vi "Step Output.vi"(8 "error in (no error)":errorcluster, 11 "IV in":refnum<class "IV.lvclass">) -> (0 "error out":errorcluster, 3 "IV out":refnum<class "IV.lvclass">)   [LabVIEW 2021, in "IV.lvclass"]
uses:
  IV.lvclass
  Libraries/Utilities/Output Value/Output Value.lvclass
  C:/Git/NHMFL_Core/Libraries/Instruments/Results/Acquired Result/Acquired Result.lvclass
  Libraries/Instruments/Instrument Driver/Instrument Driver.lvclass
  IV.lvclass/IV.ctl
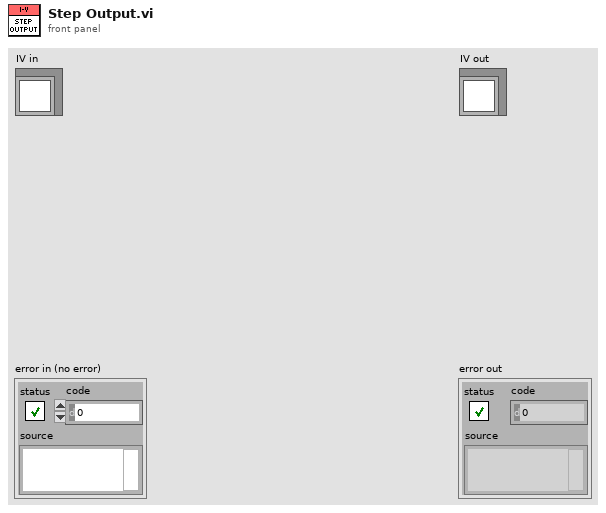
[diagram p1: front panel]
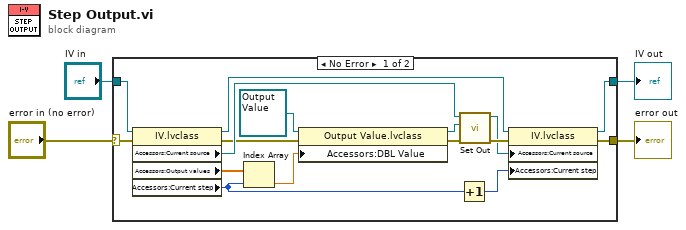
[diagram p0: block diagram]
diagram:
  n1 = case shown="No Error" "error in (no error)" {
    selector: "error in (no error)" -> [w20 w22]
    tunnel: [w14 w22] -> w3
    tunnel: [w12 w21] -> w1
    tunnel: "IV in" -> [w19 w21]
    frame No Error {
      n2 = property class="IV.lvclass"(reference=w19, error in=w20) -> (reference out=w13:refnum<class "IV.lvclass">, error out=w8:errorcluster, "Accessors:Current source "=w10:refnum<class "Instrument Driver.lvclass">, "Accessors:Output values"=w11:dbl[], "Accessors:Current step"=w5:i32)
      n3 = Index Array(array=w11, index=w5) -> (element=w16:dbl)
      n4 = property class="Output Value.lvclass"(reference=refnum<class "Output Value.lvclass"> refnum ("Output value"), error in=w8, "Accessors:DBL Value"=w16) -> (reference out=w18:refnum<class "Output Value.lvclass">, error out=w15:errorcluster)
      n5 = Increment(x=w5) -> (x+1=w6:i32)
      n6 = call-dynamic "Set Out.vi"("error in (no error)"=w15, "Output value"=w18, "Instrument Driver in"=w10) -> ("error out"=w9:errorcluster, "Instrument Driver out"=w7:refnum<class "Instrument Driver.lvclass">)  [unwired: 7 in]
      n7 = property class="IV.lvclass"(reference=w13, error in=w9, "Accessors:Current source "=w7, "Accessors:Current step"=w6) -> (reference out=w12:refnum<class "IV.lvclass">, error out=w14:errorcluster)
    }
    frame Error {
    }
  }
  "error out" <- w3
  "IV out" <- w1
